vi "CSM_serie_q_init@14.vi"(2 "Valeurs de q en abcisse":T2, 3 "Pièce":T1) -> (0 "Série Q initialisée":T2, 1 "Pièce (s)":T1)   [LabVIEW 2010, in "lv_07.lvlib"]
doc: "Si le nombre de points Nb est nul, alors la série est initialisée avec 1000 points d'un pas proportionnel à valeur de Qa"
uses:
  lv_07.lvlib
  lv_01/do_serie-c_param.ctl
  c_pi_wilson.ctl
  lv_01/lv_01.lvlib
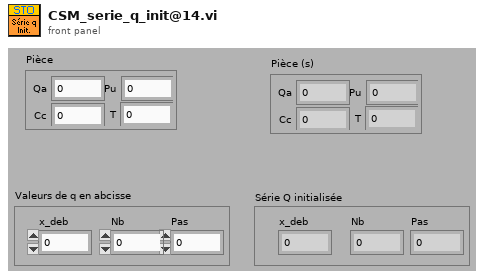
[diagram p1: front panel]
types:
  T1 = typedef "lv_07.lvlib/c_pi_wilson.ctl" = cluster{"T":dbl, "Pu":dbl, "Qa":dbl, "Cc":dbl}
  T2 = typedef "lv_01.lvlib/do_serie-c_param.ctl" = cluster{"x_deb":dbl, "Pas":dbl, "Nb":dbl}
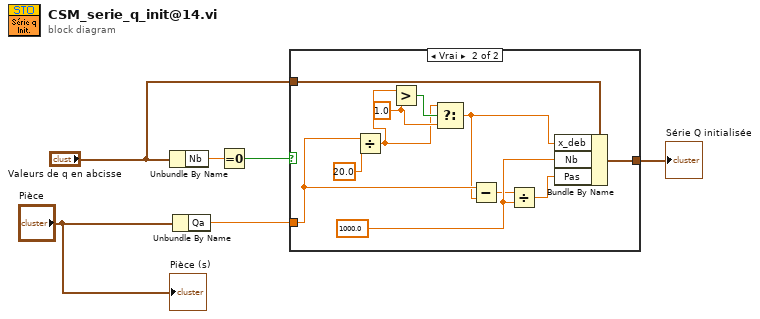
[diagram p0: block diagram]
diagram:
  n1 = Unbundle By Name("Valeurs de q en abcisse") -> ("Nb"=w4:dbl)
  n2 = Unbundle By Name("Pièce") -> ("Qa"=w6:dbl)
  n3 = Equal To 0?(x=w4) -> (x = 0?=w5:bool)
  n4 = case shown="Vrai" w5 {
    tunnel: [w7 w16] -> w2
    tunnel: w6 -> [_ w13]
    tunnel: "Valeurs de q en abcisse" -> [w7 w8]
    frame False {
    }
    frame True {
      w11 = 1.0 ("y")
      w17 = 1000.0 ("Nb")
      n5 = Divide(x=w13, y=20.0 ("q_deb")) -> (x/y=w9:dbl)
      n6 = Greater?(x=w9, y=w11) -> (0:w12:bool)
      n7 = Select(t=w9, s=w12, f=w11) -> (s? t:f=w10:dbl)
      n8 = Subtract(x=w13, y=w10) -> (x-y=w14:dbl)
      n9 = Divide(x=w14, y=w17) -> (x/y=w18:dbl)
      n10 = Bundle By Name(cluster=w8, "x_deb"=w10, "Nb"=w17, "Pas"=w18) -> (w16:T2)
    }
  }
  "Série Q initialisée" <- w2
  "Pièce (s)" <- "Pièce"
